vi "display queue to fp display_grMD.vi"() -> ()   [LabVIEW 2017]
doc: "SciScan 1.2 160622"
uses:
  <vilib>/Utility/VariantDataType/Type.ctl
  GFG/GFGnumericGet.vi
  GFG/GFGImageRefsGet.vi
  GFG/GFGDisplayRefsGet.vi
  GFG/GFGbooleanGet.vi
  GFG/GFG library.lvlib
  <vilib>/Utility/VariantDataType/VariantType.lvlib
panel:
  out "error out 2":errorcluster
  out "size(s)":i32[](array[numeric])
  out "# elements in display data queue":i32
  out "error out":errorcluster
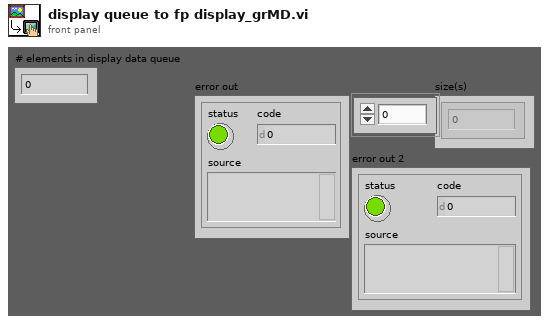
[diagram p1: front panel]
types:
  T1 = cluster{"NewVal":bool, "Event Registration Refnum":refnum<event-registration>}
  T2 = cluster{"Channel 1 small":refnum<vi>, "Channel 2 small":refnum<vi>, "Channel 3 small":refnum<vi>, "Channel 4 small":refnum<vi>, "Channel 1 large":refnum<vi>, "Channel 2 large":refnum<vi>, "Channel 3 large":refnum<vi>, "Channel 4 large":refnum<vi>, "RGB overlay":refnum<vi>, "ROI Image display":refnum<vi>, "arb line scan display":refnum<vi>, "Channel 5 large":refnum<vi>}
  T3 = typedef "IMAQ Image.ctl" = refnum<image>
  T4 = cluster{"Channel 1 small":T3, "Channel 2 small":T3, "Channel 3 small":T3, "Channel 4 small":T3, "Channel 1 large":T3, "Channel 2 large":T3, "Channel 3 large":T3, "Channel 4 large":T3, "RGB overlay":T3, "ROI Image display":T3, "arb line scan display":T3, "Channel 5 large":T3}
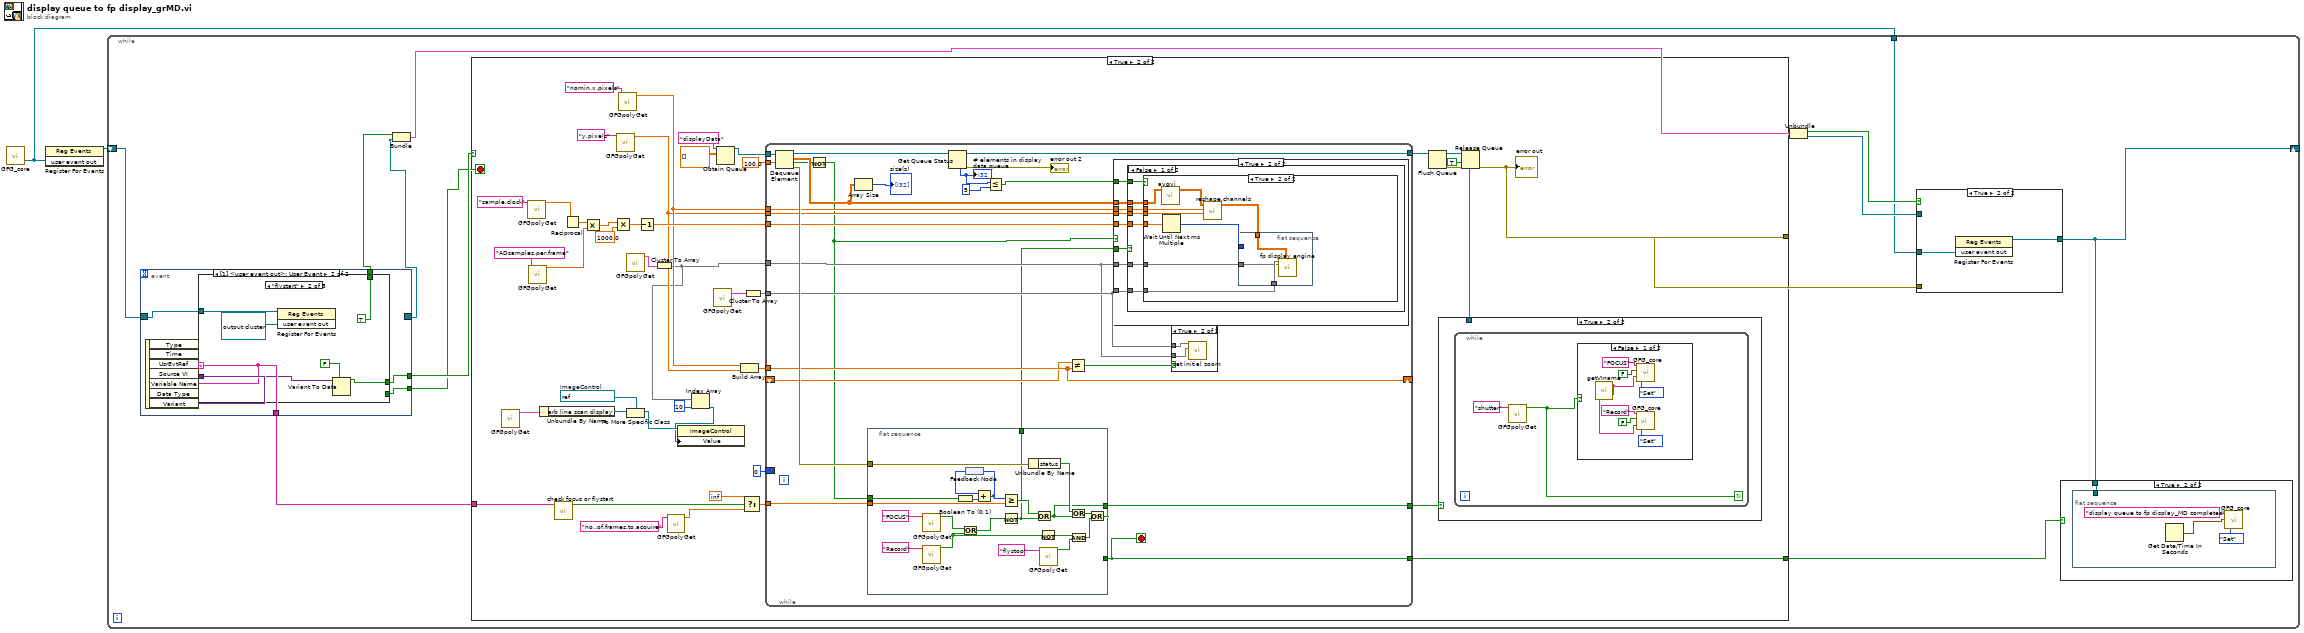
[diagram p0: block diagram]
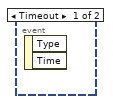
[diagram p4: hidden frame]
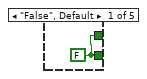
[diagram p5: hidden frame]
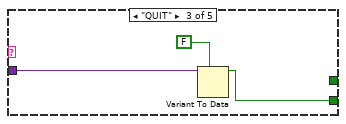
[diagram p6: hidden frame]
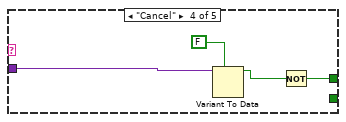
[diagram p7: hidden frame]
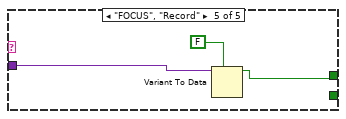
[diagram p8: hidden frame]
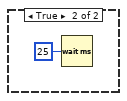
[diagram p11: hidden frame]
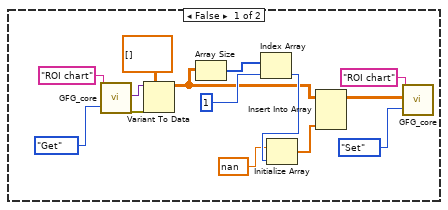
[diagram p13: hidden frame]
diagram:
  n1 = call "GFG_core.vi"() -> ("user event out"=w1:refnum<user-event>)  [unwired: 13 in, 6 out]
  n2 = register-events(w1) -> (reference out=w2:refnum<event-registration>)  [unwired: 2 in, 1 out]
  n3 = while {
    shift-right: [w4] -> _
    shift-left: w2 -> [w15]
    tunnel: w1 -> [w6]
    stop <- w13 stop-if-true
    n4 = event shown="[1] <user event out>: User Event" {
      selector: w15 -> [_ w24]
      dyn-events: [_ _] -> w11
      timeout: _ -> [_ _]
      tunnel: [_ w28] -> w14
      tunnel: [_ w27] -> w13
      tunnel: [_ w25] -> w5
      tunnel: [_ w23] -> w12
      event Timeout {
        n5 = event-data() -> ()  [unwired: 1 in, 2 out]
      }
      event User Event {
        n6 = event-data() -> ("Variable Name"=w25:string, "Variant"=w26:variant)  [unwired: 1 in, 5 out]
        n7 = case shown="\"flystart\"" w25 {
          tunnel: [w29 w33 _ w39 w43] -> w28
          tunnel: [w29 _ w36 _ _] -> w27
          tunnel: w26 -> [_ w34 w38 w41 w44]
          tunnel: w24 -> [_ w31 _ _ _]
          tunnel: [_ TRUE ("NewVal") _ _ _] -> w23
          frame "False", Default {
            w29 = FALSE ("NewVal")
          }
          frame "flystart" {
            n8 = register-events(reference=w31, refnum<user-event> refnum ("user event out")) -> ()  [unwired: 1 in, 2 out]
            n9 = Variant To Data(type=FALSE ("NewVal"), Variant=w34) -> (data=w33:bool)  [unwired: 1 in, 1 out]
          }
          frame "QUIT" {
            n10 = Variant To Data(type=FALSE ("NewVal"), Variant=w38) -> (data=w36:bool)  [unwired: 1 in, 1 out]
          }
          frame "Cancel" {
            n11 = Variant To Data(type=FALSE ("NewVal"), Variant=w41) -> (data=w40:bool)  [unwired: 1 in, 1 out]
            n12 = Not(x=w40) -> (.not. x?=w39:bool)
          }
          frame "FOCUS", "Record" {
            n13 = Variant To Data(type=FALSE ("NewVal"), Variant=w44) -> (data=w43:bool)  [unwired: 1 in, 1 out]
          }
        }
      }
    }
    n14 = Bundle("NewVal"=w12, "Event Registration Refnum"=w11) -> (w9:T1)  [unwired: 1 in]
    n15 = case shown="True" w14 {
      tunnel: [_ w67] -> w10
      tunnel: w5 -> [_ w62]
      tunnel: [_ w59] -> w3
      frame False {
      }
      frame True {
        w50 = refnum<vi> refnum  # ImageControl
        n16 = call-poly "GFGpolyGet.vi"() -> ("DisplayRefsOut(generic class)"=w52:T2)  [unwired: 10 in, 1 out]
        n17 = call-poly "GFGpolyGet.vi"("Variable Name in"="sample.clock" ("Tag in")) -> ("Numeric"=w79:dbl)  [unwired: 8 in, 2 out]
        n18 = call-poly "GFGpolyGet.vi"("Variable Name in"="ADsamples.per.frame" ("Tag in")) -> ("Numeric"=w69:dbl)  [unwired: 8 in, 2 out]
        n19 = Unbundle By Name(w52) -> ("arb line scan display"=w51:refnum<vi>)
        n20 = call "check focus or flystart.vi"("GFG variable name"=w62) -> ("Focus or flystart?"=w61:bool)  [unwired: 10 in]
        n21 = Reciprocal(x=w79) -> (1/x=w84:dbl)
        n22 = Multiply(x=w84, y=w69) -> (x*y=w83:dbl)
        n23 = Multiply(x=w83, y=1000.0 ("x")) -> (x*y=w81:dbl)
        n24 = call-poly "GFGpolyGet.vi"("Variable Name in"="y.pixels") -> ("Numeric"=w56:dbl)  [unwired: 8 in, 2 out]
        n25 = call-poly "GFGpolyGet.vi"("Variable Name in"="nomin.x.pixels") -> ("Numeric"=w57:dbl)  [unwired: 8 in, 2 out]
        n26 = call-poly "GFGpolyGet.vi"() -> ("Image Refs Out"=w74:T4)  [unwired: 10 in, 1 out]
        n27 = To More Specific Class(target class=w50, reference=w51) -> (specific class reference=w49:refnum<vi>)  [unwired: 1 in, 1 out]
        n28 = Decrement(x=w81) -> (x-1=w68:dbl)
        n29 = Cluster To Array(cluster=w74) -> (array=w47:T3[])
        n30 = call-poly "GFGpolyGet.vi"("Variable Name in"="no..of.frames.to.acquire" ("Tag in")) -> ("Numeric"=w64:dbl)  [unwired: 8 in, 2 out]
        n31 = Index Array(array=w47, index=10) -> (element=w46:T3)
        n32 = property class="ImageControl"(reference=w49, "Value"=w46) -> ()  [unwired: 1 in, 2 out]
        n33 = call-poly "GFGpolyGet.vi"() -> ("DisplayRefsOut(generic class)"=w75:T2)  [unwired: 10 in, 1 out]
        n34 = Obtain Queue(name (unnamed)="displayData", element data type=dbl[][] [] ("y backward image")) -> (queue out=w76:refnum<queue>)  [unwired: 3 in, 2 out]
        n35 = Build Array(w57, w56) -> (w55:dbl[])
        n36 = Select(t=inf, s=w61, f=w64) -> (s? t:f=w63:dbl)
        n37 = Cluster To Array(cluster=w75) -> (array=w73:refnum<vi>[])
        n38 = while {
          tunnel: [w118] -> w72
          tunnel: w63 -> [w122]
          tunnel: 100.0 -> [w106]
          tunnel: w76 -> [w120]
          tunnel: w73 -> [w117]
          tunnel: w47 -> [w111]
          tunnel: w57 -> [w104]
          tunnel: w56 -> [w109]
          tunnel: w68 -> [w116]
          tunnel: [w108] -> w60
          tunnel: [w107] -> w59
          tunnel: w55 -> [w102]
          shift-right: [w102] -> _
          shift-left: _ -> [w101]
          border: i16 0 -> [_]
          stop <- w107 stop-if-true
          n39 = Dequeue Element(queue=w120, timeout in ms (-1)=w106) -> (queue out=w119:refnum<queue>, element=w113:dbl[][], timed out?=w105:bool, error out=w121:errorcluster)  [unwired: 1 in]
          n40 = Not(x=w105) -> (.not. x?=w98:bool)
          n41 = Array Size(array=w113) -> (size(s)=→"size(s)":i32[])
          n42 = flat-sequence {
            tunnel: w122 -> [w142]
            tunnel: w121 -> [w141]
            tunnel: [w138] -> w108
            tunnel: [w137] -> w107
            tunnel: [w124] -> w99
            tunnel: w98 -> [w123]
            frame #0 {
              n43 = call-poly "GFGpolyGet.vi"("Variable Name in"="FOCUS") -> ("Boolean Value OUT"=w134:bool)  [unwired: 9 in, 1 out]
              n44 = call-poly "GFGpolyGet.vi"("Variable Name in"="Record") -> ("Boolean Value OUT"=w128:bool)  [unwired: 9 in, 1 out]
              n45 = Boolean To (0,1)(Boolean=w123) -> (0, 1=w127:i16)
              n46 = Or(x=w134, y=w128) -> (x .or. y?=w135:bool)
              n47 = feedback #1() -> (w126:i16)
              n48 = Add(x=w126, y=w127) -> (x+y=w125:i16)
              n49 = feedback-in #1(w125) -> ()
              n50 = Greater Or Equal?(x=w125, y=w142) -> (x >= y?=w140:bool)
              n51 = Not(x=w135) -> (.not. x?=w124:bool)
              n52 = Unbundle By Name(w141) -> ("status"=w143:bool)
              n53 = Or(x=w140, y=w124) -> (x .or. y?=w138:bool)
              n54 = Not(x=w128) -> (.not. x?=w130:bool)
              n55 = call-poly "GFGpolyGet.vi"("Variable Name in"="flystop") -> ("Boolean Value OUT"=w129:bool)  [unwired: 9 in, 1 out]
              n56 = Or(x=w143, y=w138) -> (x .or. y?=w139:bool)
              n57 = And(x=w130, y=w129) -> (x .and. y?=w136:bool)
              n58 = Or(x=w139, y=w136) -> (x .or. y?=w137:bool)
            }
          }
          n59 = Get Queue Status(queue=w119) -> (queue out=w118:refnum<queue>, error out=→"error out 2":errorcluster, # elements in queue=w115:i32)  [unwired: 2 in, 5 out]
          "# elements in display data queue" <- w115
          n60 = Less Or Equal?(x=w115, y=5) -> (x <= y?=w100:bool)
          n61 = Not Equal?(x=w101, y=w102) -> (x != y?=w103:bool)
          n62 = case shown="True" w98 {
            tunnel: w117 -> [_ w151]
            tunnel: w116 -> [_ w150]
            tunnel: w113 -> [_ w149]
            tunnel: w111 -> [_ w148]
            tunnel: w109 -> [_ w147]
            tunnel: w104 -> [_ w146]
            tunnel: w100 -> [_ w145]
            tunnel: w99 -> [_ w144]
            frame False {
            }
            frame True {
              n63 = case shown="False" w144 {
                tunnel: w146 -> [w158 _]
                tunnel: w147 -> [w157 _]
                tunnel: w149 -> [w156 _]
                tunnel: w151 -> [w155 _]
                tunnel: w148 -> [w154 _]
                tunnel: w150 -> [w153 _]
                tunnel: w145 -> [w152 _]
                frame False {
                  n64 = case shown="True" w152 {
                    tunnel: w158 -> [_ w181]
                    tunnel: w157 -> [_ w180]
                    tunnel: w156 -> [_ w179]
                    tunnel: w155 -> [_ w176]
                    tunnel: w154 -> [_ w175]
                    tunnel: w153 -> [_ w174]
                    frame False {
                      n65 = call "GFG_core.vi"("Variable Name in"="ROI chart", "Action"=enum16{"Init", "Set", "Get"}."Get") -> ("Variant Out"=w169:variant, "error out"=w170:errorcluster)  [unwired: 11 in, 5 out]
                      n66 = Variant To Data(error in=w170, type=sgl[][] [] ("y backward image"), Variant=w169) -> (data=w164:sgl[][])  [unwired: 1 out]
                      n67 = Array Size(array=w164) -> (size(s)=w162:i32[])
                      n68 = Index Array(array=w162, index=1) -> (element=w166:i32)
                      n69 = Initialize Array(nan, w166) -> (w163:dbl[])
                      n70 = Insert Into Array(array=w164, new element=w163) -> (w159:sgl[][])  [unwired: 2 in]
                      n71 = call "GFG_core.vi"("Variable Name in"="ROI chart", "Variant in"=w159, "Action"=enum16{"Init", "Set", "Get"}."Set") -> ()  [unwired: 10 in, 7 out]
                    }
                    frame True {
                      n72 = call "avgvi.vi"("image in"=w179) -> ("image out"=w178:sgl[][])  [unwired: 10 in]
                      n73 = Wait Until Next ms Multiple(millisecond multiple=w174) -> (millisecond timer value=w173:u32)
                      n74 = call "reshape.channels.vi"("y.pixels"=w180, "x.pixels"=w181, "element"=w178) -> ("Array"=w177:dbl[][][])  [unwired: 8 in]
                      n75 = flat-sequence {
                        tunnel: w177 -> [w184]
                        tunnel: w176 -> [w183]
                        tunnel: w175 -> [w182]
                        tunnel: w173 -> [_]
                        frame #0 {
                          n76 = call "fp display engine.vi"("channel data in"=w184, "Image Refs In"=w182, "DisplayRefsIn(generic class)"=w183) -> ()  [unwired: 9 in]
                        }
                      }
                    }
                  }
                }
                frame True {
                }
              }
            }
          }
          n77 = case shown="True" w103 {
            tunnel: w117 -> [_ w186]
            tunnel: w111 -> [_ w185]
            frame False {
            }
            frame True {
              n78 = call "set initial zoom.vi"("Image Refs In"=w185, "DisplayRefsIn(generic class)"=w186) -> ()  [unwired: 10 in]
            }
          }
        }
        n79 = Flush Queue(queue=w72) -> (queue out=w87:refnum<queue>, error out=w86:errorcluster)  [unwired: 1 in, 1 out]
        n80 = case shown="True" w60 {
          tunnel: w72 -> [_ _]
          frame False {
          }
          frame True {
            n81 = while {
              stop <- w88 continue-if-true
              n82 = call-poly "GFGpolyGet.vi"("Variable Name in"="shutter") -> ("Boolean Value OUT"=w88:bool)  [unwired: 9 in, 1 out]
              n83 = case shown="False" w88 {
                frame False {
                  n84 = call "getVIname.vi"() -> ("VI name"=w90:string)  [unwired: 19 in]
                  n85 = call "GFG_core.vi"("Variable Name in"="Record" ("Tag in"), "Variant in"=FALSE, "Source VI"=w90, "Action"=enum16{"Init", "Set", "Get"}."Set") -> ()  [unwired: 9 in, 7 out]
                  n86 = call "GFG_core.vi"("Variable Name in"="FOCUS" ("Tag in"), "Variant in"=FALSE, "Source VI"=w90, "Action"=enum16{"Init", "Set", "Get"}."Set") -> ()  [unwired: 9 in, 7 out]
                }
                frame True {
                  n87 = Wait (ms)(milliseconds to wait=u32 25) -> ()  [unwired: 1 out]
                }
              }
            }
          }
        }
        n88 = Release Queue(queue=w87, force destroy? (F)=TRUE, error in (no error)=w86) -> (error out=w67:errorcluster)  [unwired: 2 out]
        "error out" <- w67
      }
    }
    n89 = Unbundle(w9) -> ("NewVal"=w8:bool, "Event Registration Refnum"=w7:refnum<event-registration>)
    n90 = case shown="True" w8 {
      tunnel: [w20 w22] -> w4
      tunnel: w6 -> [_ w21]
      tunnel: w10 -> [_ _]
      tunnel: w7 -> [w20 _]
      frame False {
      }
      frame True {
        n91 = register-events(w21) -> (reference out=w22:refnum<event-registration>)  [unwired: 2 in, 1 out]
      }
    }
    n92 = case shown="True" w3 {
      tunnel: w4 -> [_ w16]
      frame False {
      }
      frame True {
        n93 = flat-sequence {
          tunnel: w16 -> [_]
          frame #0 {
            n94 = Get Date/Time In Seconds() -> (seconds since 1Jan1904=w17:timestamp)
            n95 = call "GFG_core.vi"("Variable Name in"="display queue to fp display_MD completed", "Variant in"=w17, "Action"=enum16{"Init", "Set", "Get"}."Set") -> ()  [unwired: 10 in, 7 out]
          }
        }
      }
    }
  }
